vi "Write file.vi"(8 "error in (no error)":errorcluster, 9 "Logging Path":path, 10 "Flicker Waveform":waveform(dbl)(graph), 11 "Metadata":string[][](array[string])) -> (0 "error out":errorcluster, 3 "file path out":path)   [LabVIEW 2014, in "Flicker.lvlib" / "Flicker Logging.lvlib"]
uses:
  Flicker Logging.lvlib
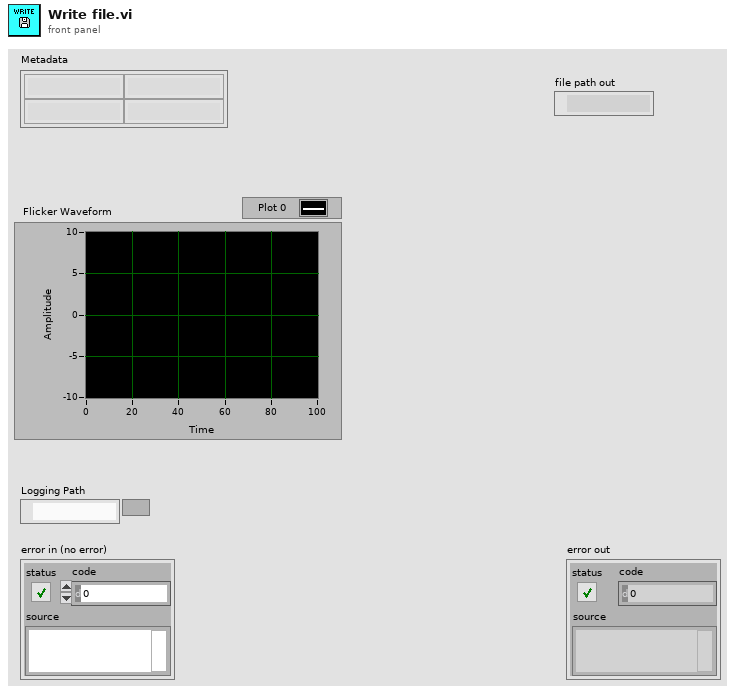
[diagram p1: front panel]
types:
  T1 = enum16{"open", "open or create", "create or replace", "create", "open (read-only)"}
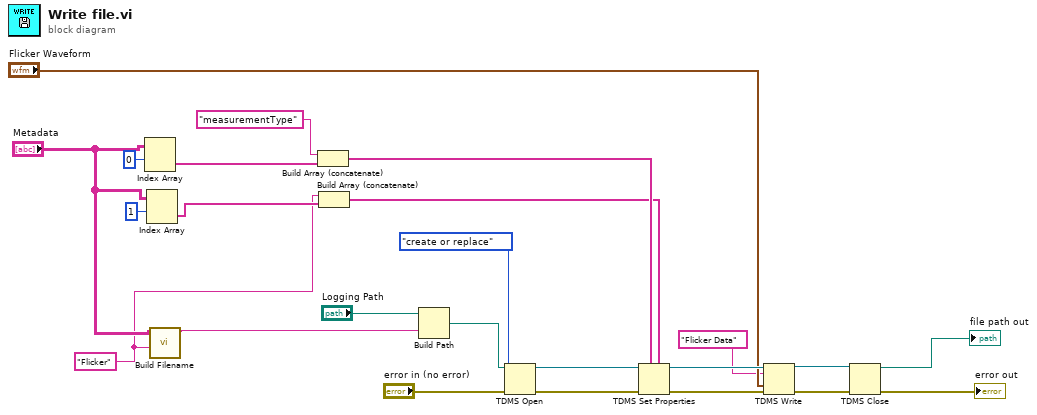
[diagram p0: block diagram]
diagram:
  w1 = "Flicker" ("Measurment Type")
  n1 = Index Array(array="Metadata", index (row)=0) -> (element=w11:string[])  [unwired: 1 in]
  n2 = Index Array(array="Metadata", index (row)=1) -> (element=w9:string[])  [unwired: 1 in]
  n3 = call "Build Filename.vi"("Measurment Type"=w1, "Metadata In"="Metadata") -> ("String"=w3:string)  [unwired: 9 in]
  n4 = Build Array (concatenate)("measurementType" ("Measurment Type"), w11) -> (w10:string[])
  n5 = Build Array (concatenate)(w1, w9) -> (w8:string[])
  n6 = Build Path(base path="Logging Path", name or relative path=w3) -> (appended path=w13:path)
  n7 = TDMS Open(8:"error in (no error)", 10:T1."create or replace" ("operation (0:open)"), 11:w13) -> (0:w18:errorcluster, 3:w19:refnum<k34>)  [unwired: 4 in]
  n8 = TDMS Set Properties(5:w8, 7:w10, 8:w18, 11:w19) -> (0:w7:errorcluster, 3:w6:refnum<k34>)  [unwired: 2 in, 2 out]
  n9 = TDMS Write(0:w6, 5:"Flicker Data" ("group name"), 9:"Flicker Waveform", 11:w7) -> (4:w24:refnum<k34>, 15:w23:errorcluster)  [unwired: 2 in, 2 out]
  n10 = TDMS Close(8:w23, 11:w24) -> (0:→"error out":errorcluster, 3:→"file path out":path)
